vi "CHD_Teleop_System_Execute.vi"(11 "Teleop Elapsed Seconds":dbl) -> ()   [LabVIEW 2019]
uses:
  <vilib>/Rock Robotics/Network Tables/NT Write Numeric Array.vi
  <vilib>/Rock Robotics/Network Tables/NT Write Boolean Array.vi
  <vilib>/Rock Robotics/WPI/ThirdParty/JAS_Junk/TrajLib/Trajectory_Library.lvlib
  <vilib>/Rock Robotics/WPI/Joystick/XBox Buttons Indexer.ctl
  <vilib>/Rock Robotics/WPI/Joystick/XBox Axes Indexer.ctl
  <vilib>/Rock Robotics/WPI/Joystick/WPI_JoystickArcadeMapping.vi
  <vilib>/Rock Robotics/Network Tables/NT Write Integer Array.vi
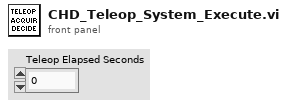
[diagram p1: front panel]
types:
  T1 = typedef "XBox Buttons Indexer.ctl" = enum16{"A", "B", "X", "Y", "Left Bumper", "Right Bumper", "Back", "Start", "Left Joystick", "Right Joystick"}
  T2 = typedef "XBox Axes Indexer.ctl" = enum16{"Left X", "Left Y", "Left Trigger", "Right Trigger", "Right X", "Right Y"}
  T3 = typedef "WPI_JoystickDevRef.ctl" = cluster{"Device":T4}
  T4 = typedef "WPI_JoystickDeviceEnum.ctl" = enum16{"USB 0", "USB 1", "USB 2", "USB 3", "USB 4", "USB 5"}
  T5 = typedef "Trajectory_Library.lvlib/DIFF_DRIVE_KINEMATICS.ctl" = cluster{"TrackWidth_Meters":dbl}
  T6 = typedef "Trajectory_Library.lvlib/CHASSIS_SPEEDS.ctl" = cluster{"vX":dbl, "vY":dbl, "vOmega":dbl}
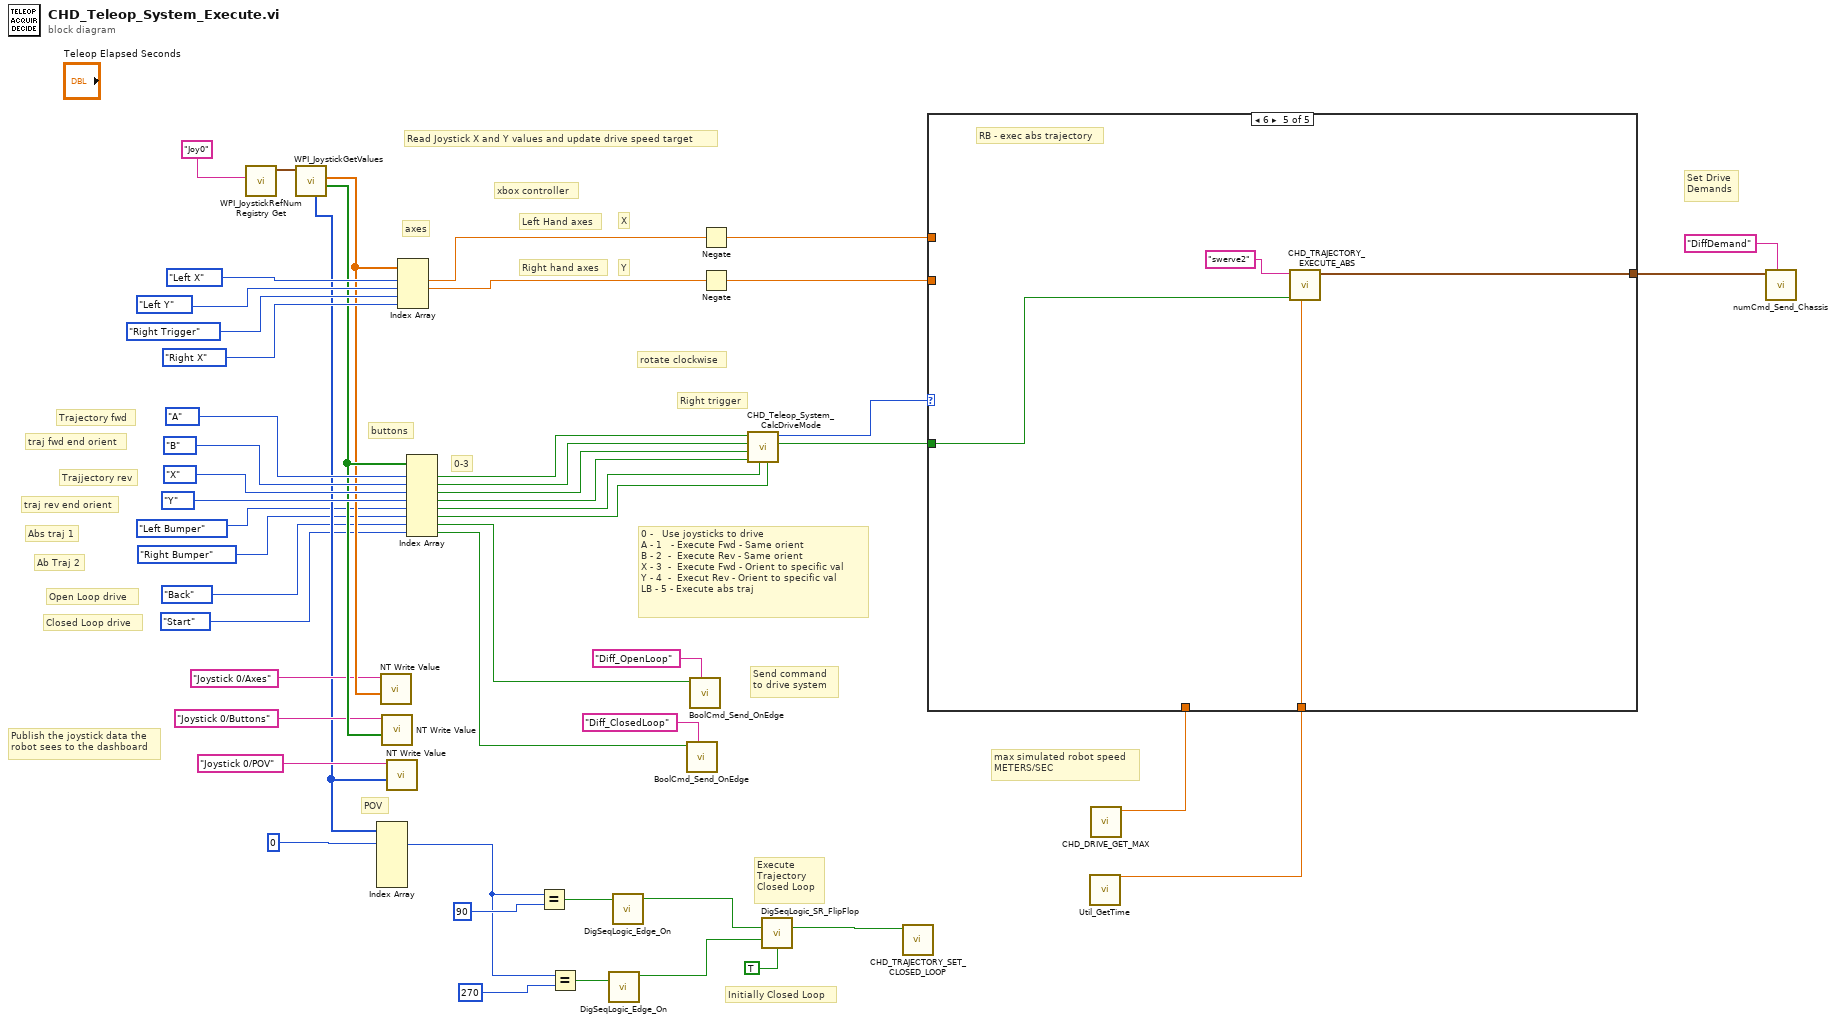
[diagram p0: block diagram]
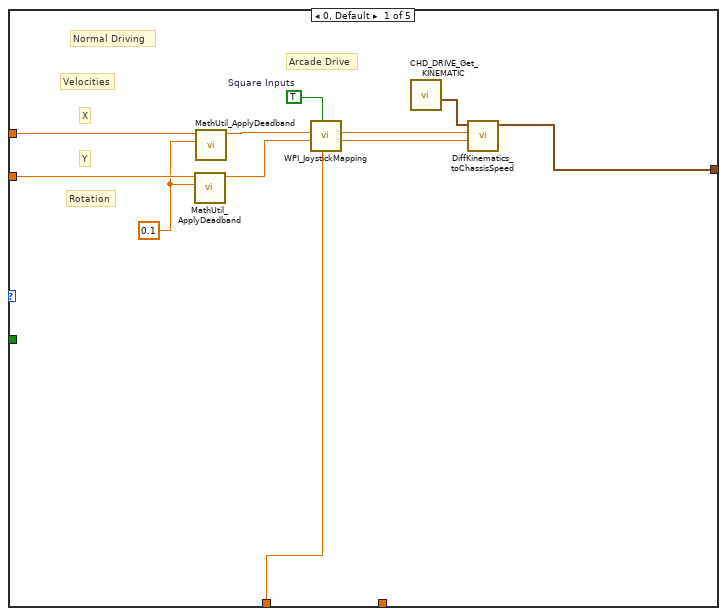
[diagram p2: hidden frame]
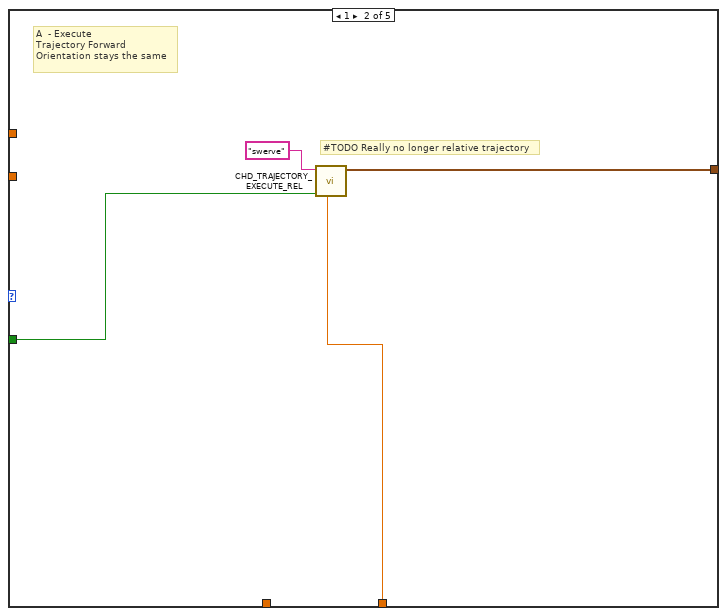
[diagram p3: hidden frame]
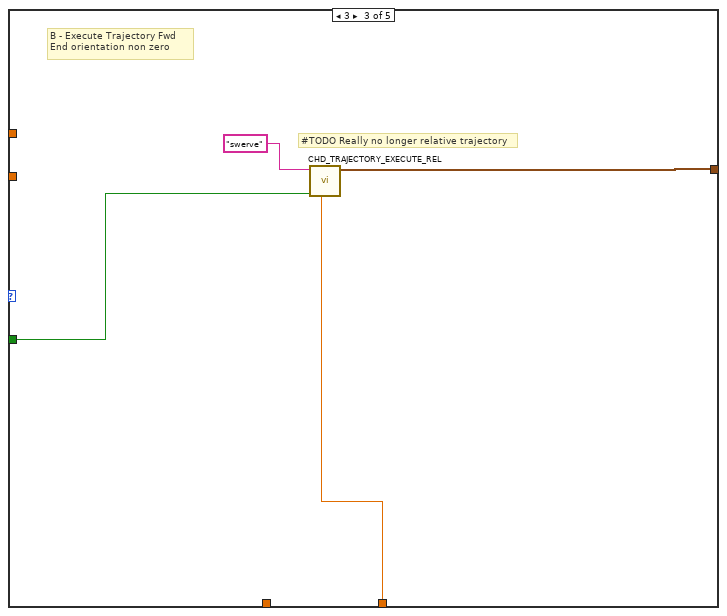
[diagram p4: hidden frame]
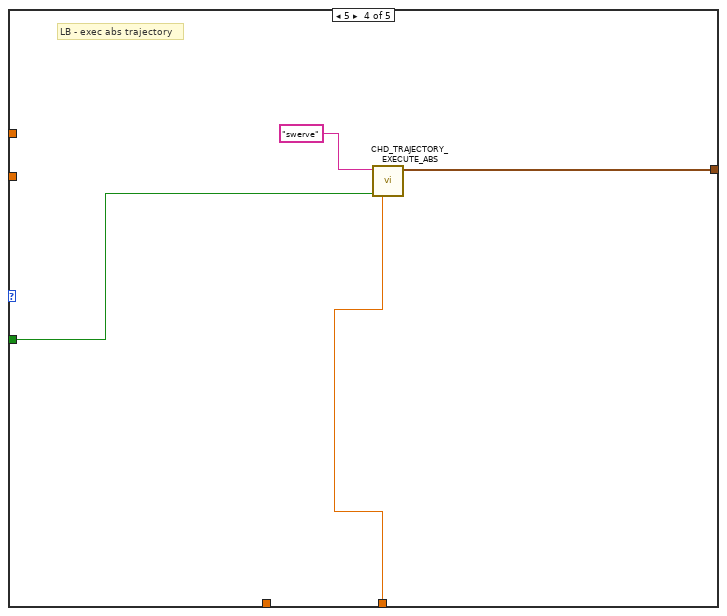
[diagram p5: hidden frame]
diagram:
  # "Send command\nto drive system"
  # "Ab Traj 2"
  # "Abs traj 1"
  # "POV"
  # "traj rev end orient"
  # "traj fwd end orient"
  # "Trajjectory rev"
  # "Closed Loop drive"
  # "Open Loop drive"
  # "Trajectory fwd"
  # "0 -   Use joysticks to drive\nA - 1   - Execute Fwd - Same orient\nB - 2  -  Execute Rev - Same orient\nX - 3  -  Execute Fwd - Orient to specific val\nY - 4  -  Execut Rev - Orient to specific val\nLB - 5 - Execute abs traj"
  # "Execute\nTrajectory\nClosed Loop"
  # "Set Drive\nDemands"
  # "Initially Closed Loop"
  # "0-3"
  # "xbox controller"
  # "Right trigger"
  # "rotate clockwise"
  # "Left Hand axes"
  # "Right hand axes"
  # "Y"
  # "X"
  # "buttons"
  # "axes"
  # "max simulated robot speed\nMETERS/SEC"
  # "Publish the joystick data the\nrobot sees to the dashboard"
  # "Read Joystick X and Y values and update drive speed target"
  n1 = call <vilib>:"WPI_JoystickRefNum Registry Get.vi"("refnum name"="Joy0") -> ("JoystickDevRef"=w27:T3)  [unwired: 1 in, 9 out]
  n2 = call <vilib>:"WPI_JoystickGetValues.vi"("JoystickDevRef"=w27) -> ("Buttons"=w31:bool[], "Axes"=w30:dbl[], "POVs"=w21:i16[])  [unwired: 6 in, 2 out]
  n3 = Index Array(array=w21, index #1=0 ("index")) -> (element #1=w17:i16)  [unwired: 5 in, 5 out]
  n4 = call-poly <vilib>:"NT Write Value.vi"("value"=w30, "name"="Joystick 0/Axes" ("Name")) -> ()  [unwired: 9 in, 1 out]
  n5 = call-poly <vilib>:"NT Write Value.vi"("value"=w31, "name"="Joystick 0/Buttons" ("Name")) -> ()  [unwired: 9 in, 1 out]
  n6 = call-poly <vilib>:"NT Write Value.vi"("value"=w21, "name"="Joystick 0/POV" ("Name")) -> ()  [unwired: 9 in, 1 out]
  n7 = Index Array(array=w30, index #1=XBox_Axes_Indexer."Left X" ("XBox Axes"), index #2=XBox_Axes_Indexer."Left Y" ("XBox Axes"), index #3=XBox_Axes_Indexer."Right Trigger" ("XBox Axes"), index #4=XBox_Axes_Indexer."Right X" ("XBox Axes")) -> (element #1=w2:dbl, element #2=w1:dbl)  [unwired: 2 out]
  n8 = Index Array(array=w31, index #1=XBox_Buttons_Indexer."A" ("XBox Buttons"), index #2=XBox_Buttons_Indexer."B" ("XBox Buttons"), index #3=XBox_Buttons_Indexer."X" ("XBox Buttons"), index #4=XBox_Buttons_Indexer."Y" ("XBox Buttons"), index #5=XBox_Buttons_Indexer."Left Bumper" ("XBox Buttons"), index #6=XBox_Buttons_Indexer."Right Bumper" ("XBox Buttons"), index #7=XBox_Buttons_Indexer."Back" ("XBox Buttons"), index #8=XBox_Buttons_Indexer."Start" ("XBox Buttons")) -> (element #1=w32:bool, element #2=w38:bool, element #3=w39:bool, element #4=w46:bool, element #5=w8:bool, element #6=w7:bool, element #7=w4:bool, element #8=w3:bool)
  n9 = Equal?(x=w17, y=i16 90) -> (x = y?=w16:bool)
  n10 = Equal?(x=w17, y=i16 270) -> (x = y?=w15:bool)
  n11 = call <vilib>:"DigSeqLogic_Edge_On.vi"("Input"=w15) -> ("On Edge"=w13:bool)  [unwired: 10 in]
  n12 = call <vilib>:"DigSeqLogic_Edge_On.vi"("Input"=w16) -> ("On Edge"=w14:bool)  [unwired: 10 in]
  n13 = call <vilib>:"BoolCmd_Send_OnEdge.vi"("Command Name"="Diff_ClosedLoop", "Value"=w3) -> ()  [unwired: 9 in, 1 out]
  n14 = call <vilib>:"BoolCmd_Send_OnEdge.vi"("Command Name"="Diff_OpenLoop", "Value"=w4) -> ()  [unwired: 9 in, 1 out]
  n15 = Negate(x=w2) -> (-x=w36:dbl)
  n16 = Negate(x=w1) -> (-x=w37:dbl)
  n17 = call "CHD_Teleop_System_CalcDriveMode.vi"("Abs Traj 2"=w7, "Abs Traj 1"=w8, "Traj Rev Follow Orient"=w46, "Traj Rev Same Orient"=w39, "Traj Fwd Follow Orient"=w38, "Traj Fwd Same Orient"=w32) -> ("Dirve Mode Changed"=w34:bool, "Drive Mode"=w33:i32)  [unwired: 4 in]
  n18 = call <vilib>:"DigSeqLogic_SR_FlipFlop.vi"("Set"=w14, "Reset"=w13, "Initial Value"=TRUE) -> ("Output"=w41:bool)  [unwired: 11 in, 1 out]
  n19 = call "CHD_TRAJECTORY_SET_CLOSED_LOOP.vi"("AUTO_CLOSED_LOOP"=w41) -> ()  [unwired: 11 in]
  n20 = call <vilib>:"Util_GetTime.vi"() -> ("FPGA_Time_Seconds"=w25:dbl)  [unwired: 9 in, 2 out]
  n21 = call "CHD_DRIVE_GET_MAX.vi"() -> ("Max Wheel Vel (Meter/Sec)"=w35:dbl)  [unwired: 11 in]
  n22 = case shown="6" w33 {
    tunnel: w37 -> [w60 _ _ _ _]
    tunnel: w35 -> [w55 _ _ _ _]
    tunnel: w34 -> [_ w65 w69 w72 w76]
    tunnel: w36 -> [w61 _ _ _ _]
    tunnel: [w51 w64 w68 w73 w77] -> w24
    tunnel: w25 -> [_ w63 w67 w71 w75]
    frame 0, Default {
      w56 = TRUE  # Square Inputs
      w59 = 0.1 ("Deadband")
      # "Normal Driving"
      # "Velocities"
      # "Rotation"
      # "Y"
      # "X"
      # "Arcade Drive"
      n23 = call <vilib>:"MathUtil_ApplyDeadband.vi"("Deadband"=w59, "Value"=w60) -> ("Result"=w57:dbl)  [unwired: 9 in]
      n24 = call <vilib>:"MathUtil_ApplyDeadband.vi"("Deadband"=w59, "Value"=w61) -> ("Result"=w58:dbl)  [unwired: 9 in]
      n25 = call-poly <vilib>:"WPI_JoystickMapping.vi"("Max Output"=w55, "Square Inputs"=w56, "Y axis value"=w57, "X axis value"=w58) -> ("Right Motor Value"=w52:dbl, "Left Motor Value"=w53:dbl)  [unwired: 6 in]
      n26 = call "CHD_DRIVE_Get_KINEMATIC.vi"() -> ("out DIFF_DRIVE_KINEMATICS"=w54:T5)  [unwired: 11 in]
      n27 = call <vilib>:"DiffKinematics_toChassisSpeed.vi"("RightVelocity"=w52, "LeftVelocity"=w53, "inDIFF_DRIVE_KINEMATICS"=w54) -> ("CHASSIS Speed"=w51:T6)  [unwired: 8 in]
    }
    frame 1 {
      # "#TODO Really no longer relative trajectory"
      # "A  - Execute\nTrajectory Forward\nOrientation stays the same"
      n28 = call "CHD_TRAJECTORY_EXECUTE_REL.vi"("Pass_Through_Time"=w63, "Init"=w65, "TrajectoryName"="swerve") -> ("Chassis Velocity Target SI"=w64:T6)  [unwired: 6 in, 2 out]
    }
    frame 3 {
      # "#TODO Really no longer relative trajectory"
      # "B - Execute Trajectory Fwd \nEnd orientation non zero"
      n29 = call "CHD_TRAJECTORY_EXECUTE_REL.vi"("Pass_Through_Time"=w67, "Init"=w69, "TrajectoryName"="swerve") -> ("Chassis Velocity Target SI"=w68:T6)  [unwired: 6 in, 2 out]
    }
    frame 5 {
      # "LB - exec abs trajectory"
      n30 = call "CHD_TRAJECTORY_EXECUTE_ABS.vi"("Pass_Through_Time"=w71, "Init"=w72, "TrajectoryName"="swerve") -> ("Chassis Velocity Target SI"=w73:T6)  [unwired: 6 in, 2 out]
    }
    frame 6 {
      # "RB - exec abs trajectory"
      n31 = call "CHD_TRAJECTORY_EXECUTE_ABS.vi"("Pass_Through_Time"=w75, "Init"=w76, "TrajectoryName"="swerve2") -> ("Chassis Velocity Target SI"=w77:T6)  [unwired: 6 in, 2 out]
    }
  }
  n32 = call <vilib>:"numCmd_Send_Chassis.vi"("Command Name"="DiffDemand", "Chassis Speeds"=w24) -> ()  [unwired: 9 in, 1 out]
